vi "Read Cycle running.vi"(11 "Temperature Control in":refnum<class "Temperature Control.lvclass">) -> (2 "Cycle running":bool, 3 "Temperature Control out":refnum<class "Temperature Control.lvclass">)   [LabVIEW 2020, in "Temperature Control.lvclass"]
uses:
  Temperature Control.lvclass
  Temperature Control.lvclass/Temperature Control.ctl
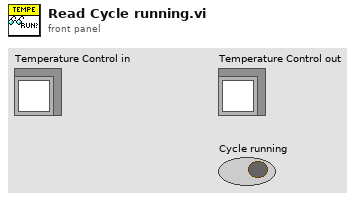
[diagram p1: front panel]
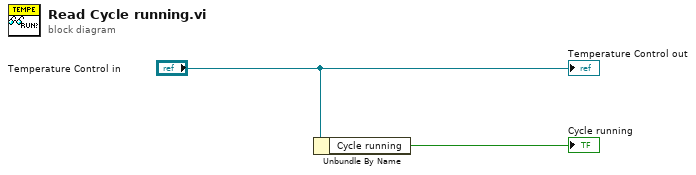
[diagram p0: block diagram]
diagram:
  n1 = Unbundle By Name("Temperature Control in") -> ("Cycle running"=→"Cycle running":bool)
  "Temperature Control out" <- "Temperature Control in"
